vi "SettingsManager.vi"(8 "error in (no error)":errorcluster) -> (0 "error out":errorcluster)   [LabVIEW 2012]
doc: "VI sets analysis parameters to FG."
uses:
  Signal/#TD_SignalStorageCommand.ctl
  #TD_AnalysisSettings.ctl
  <vilib>/addons/_Advanced Signal Processing/NI_AdvSigProcWA.lvlib
panel:
  in  "Falka":T1(ring)
  out "Wav_Prev":T2(graph)
  in  "Analizowany sygnał":i32(ring)
  in  "Ilość poziomów dekompozycji":i32
  in  "Używane falki":T3(array[ring])
  in  "Stop Button":bool
  in  "OK Button":bool
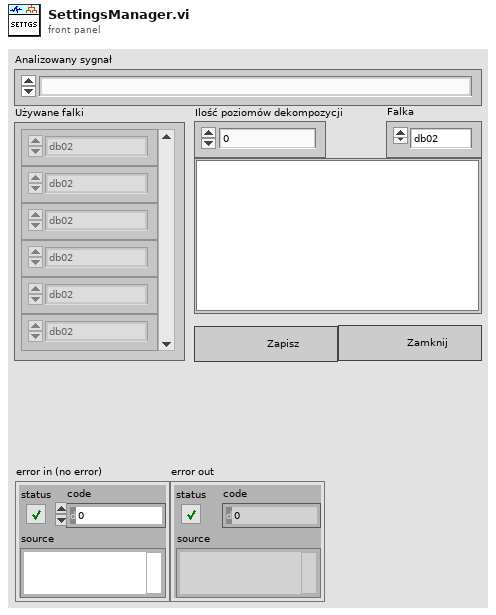
[diagram p1: front panel]
types:
  T1 = enum16{"db02", "db03", "db04", "db05", "db06", "db07", "db08", "db09", "db10", "db11", "db12", "db13", "db14", "Haar", "bior1_3", "bior1_5", "bior2_2", "bior2_4", "bior2_6", "bior2_8", "bior3_1", "bior3_3", "bior3_5", "bior3_7", "bior3_9", "bior4_4 (FBI)", "bior5_5", "bior6_8", "coif1", "coif2", "coif3", "coif4", "coif5", "sym2", "sym3", "sym4", "sym5", "sym6", "sym7", "sym8"}
  T2 = cluster{"t0":dbl, "dt":dbl, "wavelet function":dbl[]}[]
  T3 = enum16{"db02", "db03", "db04", "db05", "db06", "db07", "db08", "db09", "db10", "db11", "db12", "db13", "db14", "Haar", "bior1_3", "bior1_5", "bior2_2", "bior2_4", "bior2_6", "bior2_8", "bior3_1", "bior3_3", "bior3_5", "bior3_7", "bior3_9", "bior4_4 (FBI)", "bior5_5", "bior6_8", "coif1", "coif2", "coif3", "coif4", "coif5", "sym2", "sym3", "sym4", "sym5", "sym6", "sym7", "sym8"}[]
  T4 = typedef "#TD_SignalStorageCommand.ctl" = enum16{"Reset_Storage", "Add_Signal", "Insert_Signal", "Del_Signal", "Replace_Signal", "Get_Signal", "Get_Signal_List", "Change_Signal_Name", "Change_Signal_Descr"}
  T5 = typedef "#TD_AnalysisSettings.ctl" = cluster{"DecompLevel":i32, "WaveletsToUse":enum16{"db02", "db03", "db04", "db05", "db06", "db07", "db08", "db09", "db10", "db11", "db12", "db13", "db14", "Haar", "bior1_3", "bior1_5", "bior2_2", "bior2_4", "bior2_6", "bior2_8", "bior3_1", "bior3_3", "bior3_5", "bior3_7", "bior3_9", "bior4_4 (FBI)", "bior5_5", "bior6_8", "coif1", "coif2", "coif3", "coif4", "coif5", "sym2", "sym3", "sym4", "sym5", "sym6", "sym7", "sym8"}[], "SignalToAnalysisNb":i32}
  T6 = cluster{"t0":dbl, "dt":dbl, "wavelet function":dbl[]}
  T7 = cluster{"t0":dbl, "dt":dbl, "scaling function":dbl[]}
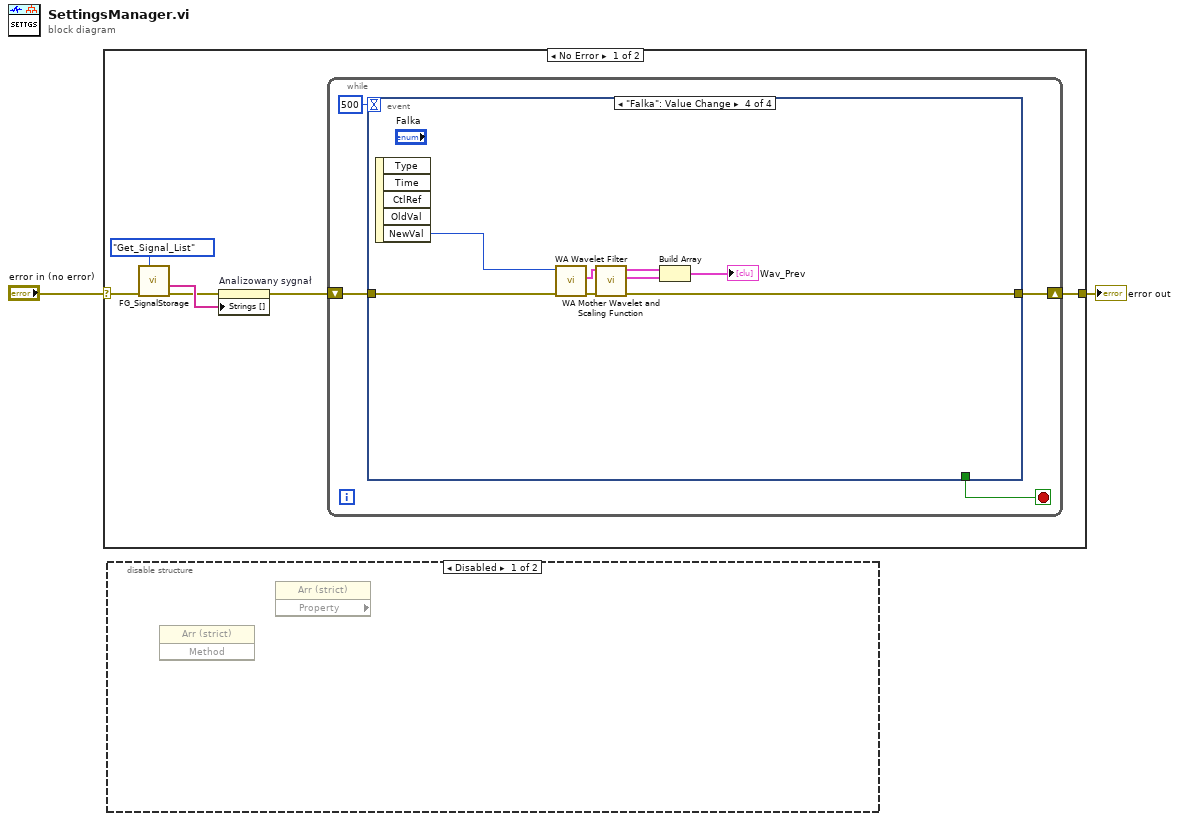
[diagram p0: block diagram]
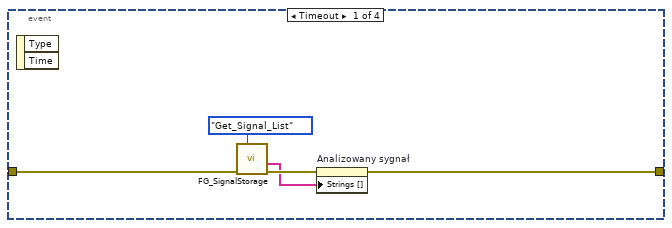
[diagram p3: hidden frame]
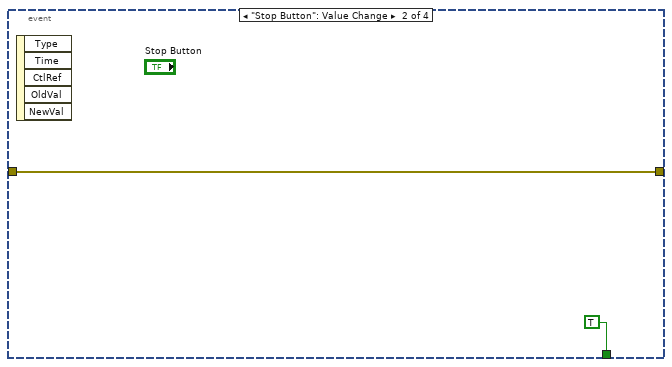
[diagram p4: hidden frame]
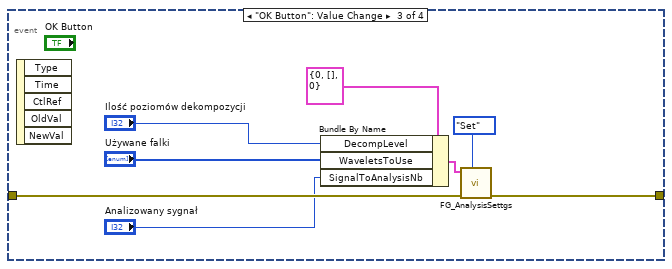
[diagram p5: hidden frame]
diagram:
  n1 = case shown="No Error" "error in (no error)" {
    selector: "error in (no error)" -> [w7 w36]
    tunnel: [w8 w36] -> w1
    frame No Error {
      n2 = call "FG_SignalStorage.vi"("Command"=#TD_SignalStorageCommand."Get_Signal_List", "error in (no error)"=w7) -> ("error out"=w4:errorcluster, "Signal_List"=w5:string[])  [unwired: 7 in, 1 out]
      n3 = property on="Analizowany sygnał" class="Ring (strict)"(error in=w4, "Strings []"=w5) -> (error out=w3:errorcluster)  [unwired: 1 in, 1 out]
      n4 = while {
        shift-right: [w11] -> w8
        shift-left: w3 -> [w12]
        stop <- w10 stop-if-true
        n5 = event shown="[3] \"Falka\": Value Change" {
          selector: _ -> [_ _ _ _]
          dyn-events: _ -> [_ _ _ _]
          timeout: 500 -> [_ _ _ _]
          tunnel: w12 -> [w14 w19 w27 w29]
          tunnel: [w13 w19 w26 w28] -> w11
          tunnel: [_ TRUE _ _] -> w10
          event Timeout {
            n6 = event-data() -> ()  [unwired: 1 in, 2 out]
            n7 = call "FG_SignalStorage.vi"("Command"=#TD_SignalStorageCommand."Get_Signal_List", "error in (no error)"=w14) -> ("error out"=w17:errorcluster, "Signal_List"=w16:string[])  [unwired: 7 in, 1 out]
            n8 = property on="Analizowany sygnał" class="Ring (strict)"(error in=w17, "Strings []"=w16) -> (error out=w13:errorcluster)  [unwired: 1 in, 1 out]
          }
          event "Stop Button": Value Change {
            n9 = event-data() -> ()  [unwired: 1 in, 5 out]
          }
          event "OK Button": Value Change {
            n10 = event-data() -> ()  [unwired: 1 in, 5 out]
            n11 = Bundle By Name(cluster=T5 {"DecompLevel"=0, "WaveletsToUse"=[], "SignalToAnalysisNb"=0} ("Settings"), "DecompLevel"="Ilość poziomów dekompozycji", "WaveletsToUse"="Używane falki", "SignalToAnalysisNb"="Analizowany sygnał") -> (w22:T5)
            n12 = call "FG_AnalysisSettgs.vi"("Command"=enum16{"Set", "Get", "Reset"}."Set", "error in (no error)"=w27, "Settings"=w22) -> ("error out"=w26:errorcluster)  [unwired: 7 in, 1 out]
          }
          event "Falka": Value Change {
            n13 = event-data() -> ("NewVal"=w30:T1)  [unwired: 1 in, 4 out]
            n14 = call <vilib>:"WA Wavelet Filter.vi"("error in (no error)"=w29, "wavelet"=w30) -> ("error out"=w34:errorcluster, "analysis filters"=w33:cluster{"lowpass":dbl[], "highpass":dbl[]})  [unwired: 6 in, 2 out]
            n15 = call <vilib>:"WA Mother Wavelet and Scaling Function.vi"("error in (no error)"=w34, "filters"=w33) -> ("error out"=w28:errorcluster, "mother wavelet function info"=w31:T6, "scaling function info"=w32:T7)  [unwired: 7 in]
            n16 = Build Array(w32, w31) -> (→"Wav_Prev":T2)
          }
        }
      }
    }
    frame Error {
    }
  }
  "error out" <- w1
  n17 = disable-structure shown="Disabled" {
    frame Disabled {
      n18 = invoke class="Arr (strict)" method=#-1() -> ()  [unwired: 3 in, 3 out]
      n19 = property class="Arr (strict)" props=[]() -> ()  [unwired: 2 in, 3 out]
    }
    frame Enabled {
    }
  }
